vi "Set XScale.vi"(8 "error in (no error)":errorcluster caption="entrée d'erreur (pas d'erreur)", 11 "UV-VIS en entrée":refnum<class "UV-VIS.lvclass">) -> (0 "error out":errorcluster caption="sortie d'erreur", 3 "UV-VIS en sortie":refnum<class "UV-VIS.lvclass">)   [LabVIEW 2015, in "UV-VIS.lvclass"]
uses:
  UV-VIS.lvclass
  Detector.lvclass
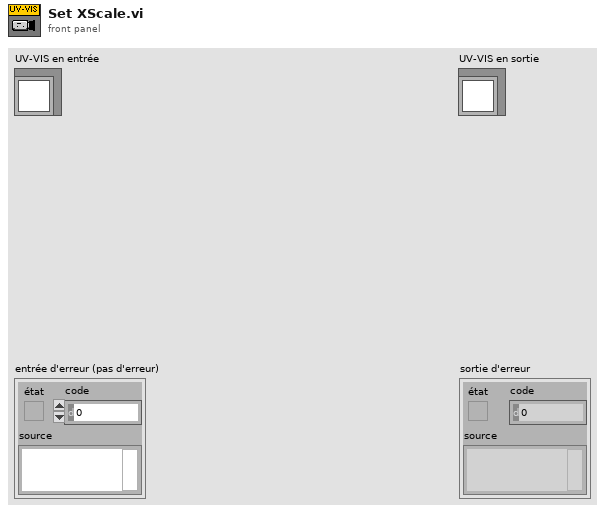
[diagram p1: front panel]
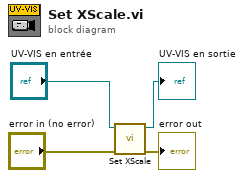
[diagram p0: block diagram]
diagram:
  n1 = call-parent "Set XScale.vi"("error in (no error)"="error in (no error)", "Detector en entrée"="UV-VIS en entrée") -> ("error out"=→"error out":errorcluster, "Detector en sortie"=→"UV-VIS en sortie":refnum<class "UV-VIS.lvclass">)  [unwired: 8 in]
